vi "demarcate_PicoScope6000ExampleBlockAdvancedTrigger.vi"() -> ()   [LabVIEW 2020]
uses:
  ps6000.dll
panel:
  in  "文件路径（使用对话框）":path
  out "最大索引":i32
  out "数组":i32[](array[numeric])
  in  "Aux. Trigger Properties":T1 {"Direction" items=["Above / Inside", "Below / Outside", "Rising / Enter", "Falling / Exit", "Rising or Falling / Enter or Exit", "Above Lower", "Below Lower", "Rising Lower", "Falling Lower", "Positive Runt", "Negative Runt"]; "Threshold Mode" items=["Level", "Window"]}
  out "Channel A":i16[](graph)
  out "Channel A Max ADC value":i16
  in  "Channel A Settings":T2={"Enabled"=TRUE, "Coupling"=1, "Range"=8, "Analogue Offset"=0.0, "Bandwidth"=0} {"Bandwidth" items=["Full", "20 MHz"]; "Range" items=["10 mV", "20 mV", "50 mV", "100 mV", "200 mV", "500 mV", "1 V", "2 V", "5 V", "10 V", "20 V", "50 V ", "100 V"]; "Coupling" items=["AC", "DC 1 MOhm", "DC 50 Ohm"]}
  in  "Auto Trigger (ms)":i32
  in  "Trigger Delay":u32
  in  "Trigger Conditions":T3={"Channel A"=FALSE, "Channel B"=FALSE, "Channel C"=TRUE, "Channel D"=FALSE, "Aux"=FALSE, "PWQ"=TRUE, "Condition Logic"=0, "Ext"=FALSE} {"Condition Logic" items=["AND", "OR", "XOR"]}
  in  "Acquisition Settings":T4={"preTriggerSamples"=2500, "postTriggerSamples"=10000, "timebase"=1, "Down-Sample Mode"=0, "Down Sample Ratio"=1, "Four Channel Device"=TRUE, "Oversample"=1} {"Down Sample Ratio" min=1 step=1; "Down-Sample Mode" items=["None"=0, "Aggregate"=1, "Average"=2, "Decimate"=4, "Distribution"=8]}
  in  "stop":bool
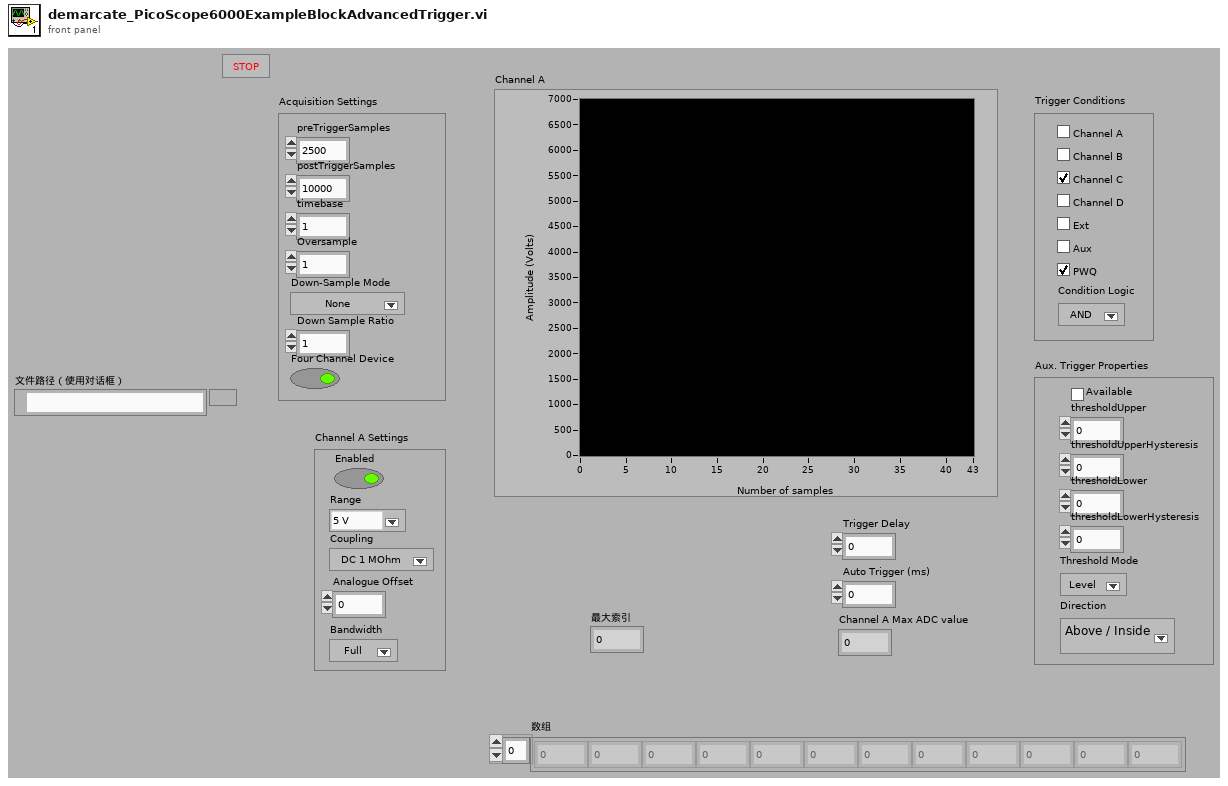
[diagram p1: front panel]
types:
  T1 = cluster{"thresholdUpper":i16, "thresholdUpperHysteresis":u16, "thresholdLower":i16, "thresholdLowerHysteresis":u16, "Threshold Mode":i32, "Direction":i32, "Available":bool}
  T2 = cluster{"Enabled":bool, "Coupling":u32, "Range":u32, "Analogue Offset":sgl, "Bandwidth":u32}
  T3 = cluster{"Channel A":bool, "Channel B":bool, "Channel C":bool, "Channel D":bool, "Aux":bool, "PWQ":bool, "Condition Logic":u16, "Ext":bool}
  T4 = cluster{"preTriggerSamples":u32, "postTriggerSamples":u32, "timebase":u32, "Down-Sample Mode":i32, "Down Sample Ratio":u32, "Four Channel Device":bool, "Oversample":i16}
  T5 = cluster{"Enabled":bool, "Coupling":i32, "Range":u16, "Analogue Offset":sgl, "Bandwidth":i32}
  T6 = cluster{"Channel D Buffer":i16[], "Channel C Buffer":i16[], "Channel B Buffer":i16[], "Channel A Buffer":i16[]}
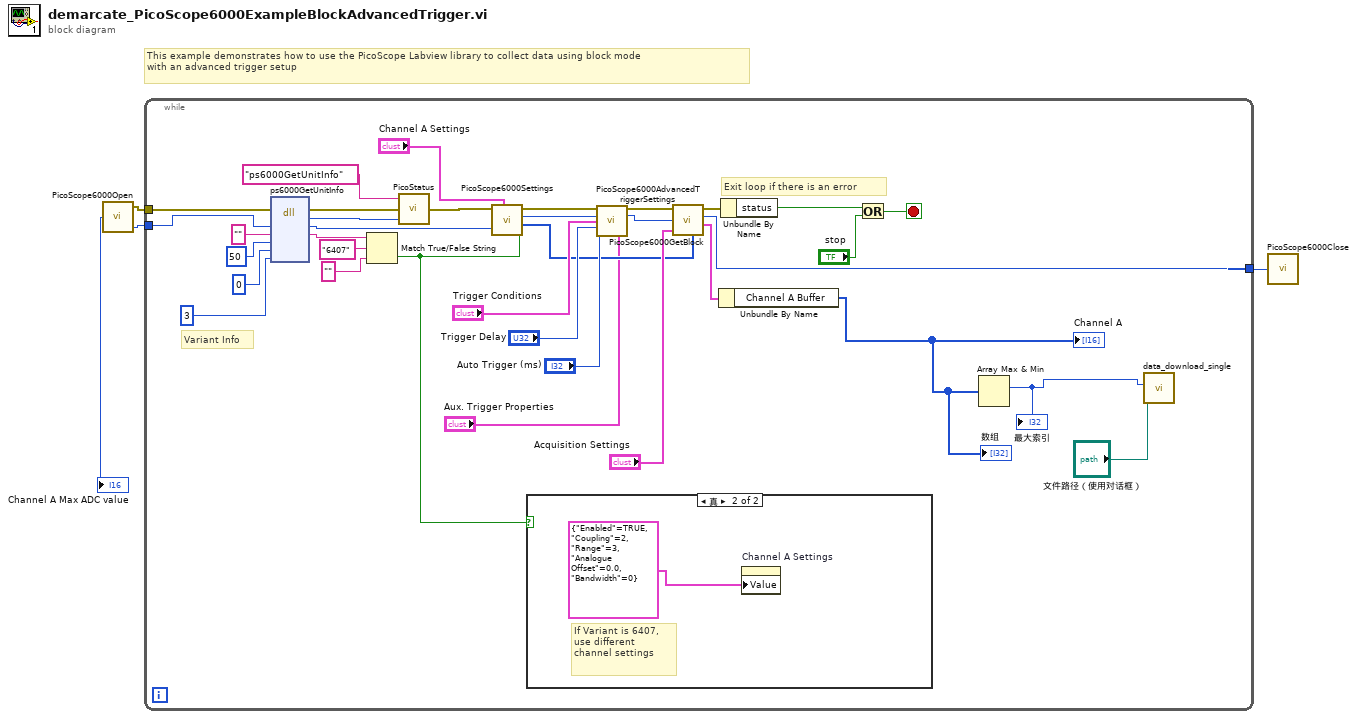
[diagram p0: block diagram]
diagram:
  # "This example demonstrates how to use the PicoScope Labview library to collect data using block mode\nwith an advanced trigger setup"
  n1 = call "PicoScope6000Open.vi"() -> ("handle"=w3:i16, "Max Adc value"=→"Channel A Max ADC value":i16, "error out"=w4:errorcluster)  [unwired: 3 in, 1 out]
  n2 = while {
    tunnel: w3 -> [w33]
    tunnel: [w35] -> w2
    tunnel: w4 -> [w34]
    stop <- w39 stop-if-true
    # "Variant Info"
    # "Exit loop if there is an error"
    n3 = dll-call lib="PS6000.dll" fn="ps6000GetUnitInfo"(error in=w34, "handle"=w33, "string"="", "stringLength"=i16 50, "reqSize"=0, "info"=i16 3) -> (error out=w26:errorcluster, "PICO_STATUS"=w25:u32, "handle"=w23:i16, "string"=w21:string)  [unwired: 5 in, 1 out]
    n4 = Match True/False String(2:"" ("false string"), 3:"6407" ("true string"), 4:w21) -> (0:w11:bool)  [unwired: 1 out]
    n5 = call "PicoStatus.vi"("PICO STATUS"=w25, "error in"=w26, "source"="ps6000GetUnitInfo") -> ("error out"=w24:errorcluster)
    n6 = call "PicoScope6000Settings.vi"("PS6407?"=w11, "Channel A Settings"="Channel A Settings", "handle in"=w23, "error in"=w24) -> ("Enabled array"=w9:i16[], "handle out"=w17:i16, "error out"=w19:errorcluster)  [unwired: 5 in]
    n7 = case shown="真" w11 {
      frame False {
      }
      frame True {
        # "If Variant is 6407,\nuse different \nchannel settings"
        n8 = property on="Channel A Settings" class="Clust (严格)"("Value"=T5 {"Enabled"=TRUE, "Coupling"=2, "Range"=3, "Analogue Offset"=0.0, "Bandwidth"=0} ("Channel A Settings")) -> ()  [unwired: 2 in, 2 out]
      }
    }
    n9 = call "PicoScope6000AdvancedTriggerSettings.vi"("error in"=w19, "handle in"=w17, "Trigger Conditions"="Trigger Conditions", "Trigger Delay"="Trigger Delay", "Auto Trigger (ms)"="Auto Trigger (ms)", "Aux. Trigger Properties"="Aux. Trigger Properties") -> ("error out"=w18:errorcluster, "handle out"=w16:i16)  [unwired: 8 in]
    n10 = call "PicoScope6000GetBlock.vi"("error in"=w18, "handle in"=w16, "Acquisition Settings"="Acquisition Settings", "Enabled array"=w9) -> ("error out"=w36:errorcluster, "handle out"=w35:i16, "Buffers (Max or non-aggregated)"=w10:T6)  [unwired: 1 in, 3 out]
    n11 = Unbundle By Name(w10) -> ("Channel A Buffer"=w7:i16[])
    "Channel A" <- w7
    "数组" <- w7
    n12 = Unbundle By Name(w36) -> ("status"=w38:bool)
    n13 = Or(x=w38, y="stop") -> (x .or. y?=w39:bool)
    n14 = Array Max & Min(array=w7) -> (max index (indices)=w6:i32)  [unwired: 3 out]
    "最大索引" <- w6
    n15 = call "data_download_single.vi"("文件路径（使用对话框）"="文件路径（使用对话框）", "数值"=w6) -> ()  [unwired: 10 in]
  }
  n16 = call "PicoScope6000Close.vi"("handle"=w2) -> ()
